vi "Detrended Amplitude.vi"(4 "location":dbl[](array[numeric]), 5 "Amplitude":dbl[](array[numeric]), 7 "Trend":cluster{"Ramp Pattern":dbl[], "X":dbl[]}) -> (3 "detrended amplitude":dbl[](array[numeric]))   [LabVIEW 2017]
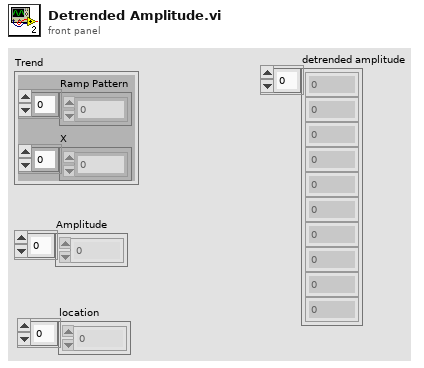
[diagram p1: front panel]
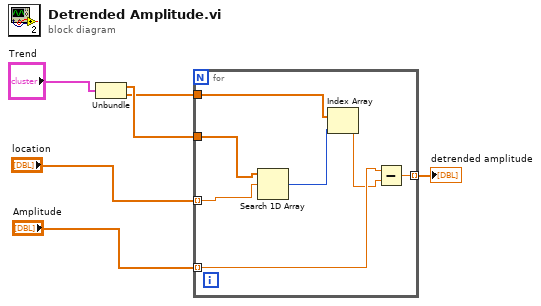
[diagram p0: block diagram]
diagram:
  n1 = Unbundle("Trend") -> ("Ramp Pattern"=w4:dbl[], "X"=w3:dbl[])
  n2 = for {
    tunnel: "location" -> [w12] mode=indexing
    tunnel: w4 -> [w13]
    tunnel: w3 -> [w10]
    tunnel: "Amplitude" -> [w9] mode=indexing
    tunnel: [w7] -> w1 mode=indexing
    n3 = Search 1D Array(1D array=w13, element=w12) -> (index of element=w11:i32)  [unwired: 1 in]
    n4 = Index Array(array=w10, index=w11) -> (element=w8:dbl)
    n5 = Subtract(x=w9, y=w8) -> (x-y=w7:dbl)
  }
  "detrended amplitude" <- w1
